vi "_logging_set_parameter.vi"(7 "Logging Parameter":T1, 8 "error in":errorcluster caption="error in (no error)", 9 "String parameter (\"\")":string, 10 "Int32 parameter (0)":i32, 11 "Logging params in":variant) -> (0 "error out":errorcluster, 3 "Logging params out":variant)   [LabVIEW 2022 SP3, in "hmp4000_rsidr_core.lvlib"]
uses:
  hmp4000_rsidr_core.lvlib
  _type_Logging_Parameter.ctl
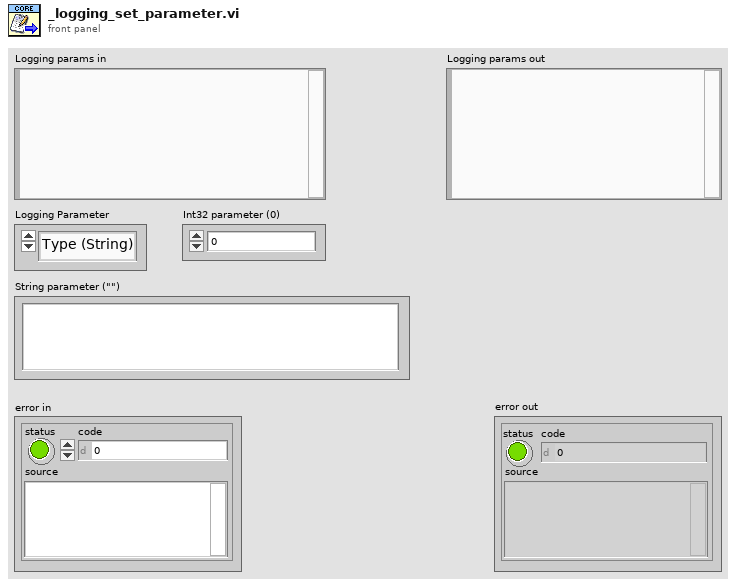
[diagram p1: front panel]
types:
  T1 = typedef "hmp4000_rsidr_core.lvlib/_type_Logging_Parameter.ctl" = enum16{"Type (String)", "SessionAlias(String)", "FormatString (String)", "UDPconectionID (I32)", "UDPlocalPort (I32)", "UDPremotePort (I32)", "UDPremoteHost (String)", "FILEmode (I32)", "FILEpath (String)", "FILEopenID (I32)", "DataMaxLogLen (I32)"}
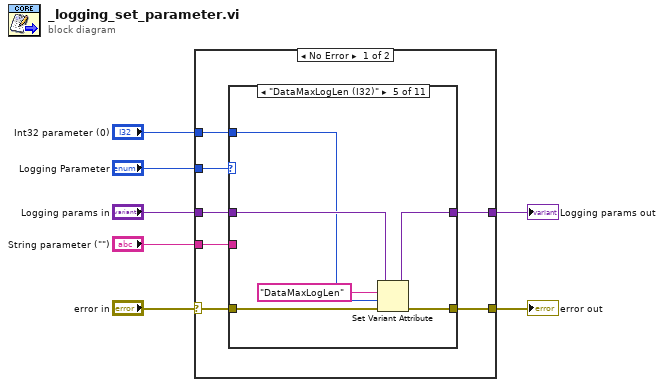
[diagram p0: block diagram]
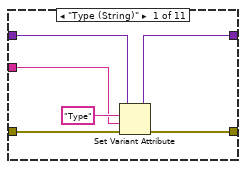
[diagram p2: hidden frame]
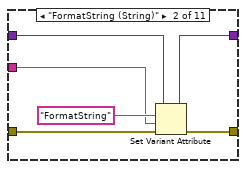
[diagram p3: hidden frame]
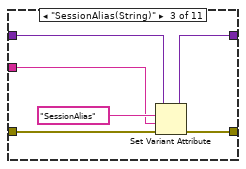
[diagram p4: hidden frame]
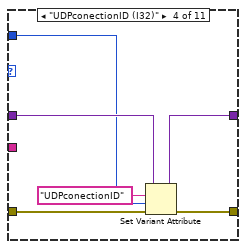
[diagram p5: hidden frame]
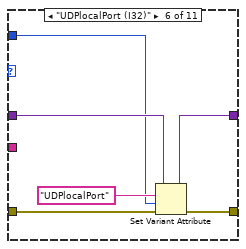
[diagram p6: hidden frame]
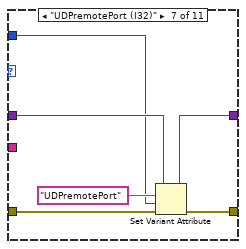
[diagram p7: hidden frame]
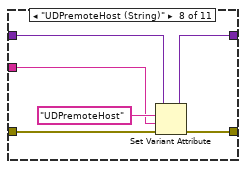
[diagram p8: hidden frame]
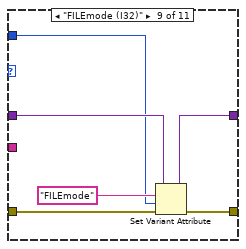
[diagram p9: hidden frame]
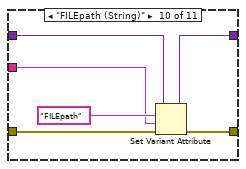
[diagram p10: hidden frame]
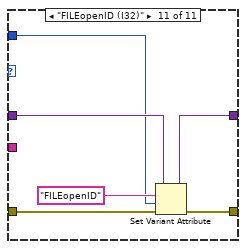
[diagram p11: hidden frame]
diagram:
  n1 = case shown="No Error" "error in" {
    selector: "error in" -> [w14 w82]
    tunnel: [w11 w82] -> w6
    tunnel: "Logging params in" -> [w13 w81]
    tunnel: [w12 w81] -> w4
    tunnel: "Int32 parameter (0)" -> [w10 _]
    tunnel: "Logging Parameter" -> [w9 _]
    tunnel: "String parameter (\"\")" -> [w8 _]
    frame No Error {
      n2 = case shown="\"DataMaxLogLen (I32)\"" w9 {
        tunnel: w14 -> [w20 w26 w32 w38 w44 w50 w56 w62 w68 w74 w80]
        tunnel: [w18 w24 w30 w36 w42 w48 w54 w60 w66 w72 w78] -> w11
        tunnel: w13 -> [w17 w23 w29 w35 w41 w47 w53 w59 w65 w71 w77]
        tunnel: w10 -> [_ _ _ w33 w39 w45 w51 _ w63 _ w75]
        tunnel: [w16 w22 w28 w34 w40 w46 w52 w58 w64 w70 w76] -> w12
        tunnel: w8 -> [w15 w21 w27 _ _ _ _ w57 _ w69 _]
        frame "Type (String)" {
          n3 = Set Variant Attribute(Variant=w17, name="Type", value=w15, error in=w20) -> (Variant out=w16:variant, error out=w18:errorcluster)  [unwired: 1 out]
        }
        frame "FormatString (String)" {
          n4 = Set Variant Attribute(Variant=w23, name="FormatString", value=w21, error in=w26) -> (Variant out=w22:variant, error out=w24:errorcluster)  [unwired: 1 out]
        }
        frame "SessionAlias(String)" {
          n5 = Set Variant Attribute(Variant=w29, name="SessionAlias", value=w27, error in=w32) -> (Variant out=w28:variant, error out=w30:errorcluster)  [unwired: 1 out]
        }
        frame "UDPconectionID (I32)" {
          n6 = Set Variant Attribute(Variant=w35, name="UDPconectionID", value=w33, error in=w38) -> (Variant out=w34:variant, error out=w36:errorcluster)  [unwired: 1 out]
        }
        frame "DataMaxLogLen (I32)" {
          n7 = Set Variant Attribute(Variant=w41, name="DataMaxLogLen", value=w39, error in=w44) -> (Variant out=w40:variant, error out=w42:errorcluster)  [unwired: 1 out]
        }
        frame "UDPlocalPort (I32)" {
          n8 = Set Variant Attribute(Variant=w47, name="UDPlocalPort", value=w45, error in=w50) -> (Variant out=w46:variant, error out=w48:errorcluster)  [unwired: 1 out]
        }
        frame "UDPremotePort (I32)" {
          n9 = Set Variant Attribute(Variant=w53, name="UDPremotePort", value=w51, error in=w56) -> (Variant out=w52:variant, error out=w54:errorcluster)  [unwired: 1 out]
        }
        frame "UDPremoteHost (String)" {
          n10 = Set Variant Attribute(Variant=w59, name="UDPremoteHost", value=w57, error in=w62) -> (Variant out=w58:variant, error out=w60:errorcluster)  [unwired: 1 out]
        }
        frame "FILEmode (I32)" {
          n11 = Set Variant Attribute(Variant=w65, name="FILEmode", value=w63, error in=w68) -> (Variant out=w64:variant, error out=w66:errorcluster)  [unwired: 1 out]
        }
        frame "FILEpath (String)" {
          n12 = Set Variant Attribute(Variant=w71, name="FILEpath", value=w69, error in=w74) -> (Variant out=w70:variant, error out=w72:errorcluster)  [unwired: 1 out]
        }
        frame "FILEopenID (I32)" {
          n13 = Set Variant Attribute(Variant=w77, name="FILEopenID", value=w75, error in=w80) -> (Variant out=w76:variant, error out=w78:errorcluster)  [unwired: 1 out]
        }
      }
    }
    frame Error {
    }
  }
  "error out" <- w6
  "Logging params out" <- w4
